vi "Device to String.vi"(11 "Devices":T1[](array[typedef])) -> (3 "delimited string":string)   [LabVIEW 2019, in "DAQmx.lvclass"]
uses:
  DAQmx.lvclass
  typedefs/DeviceInfo--Cluster.ctl
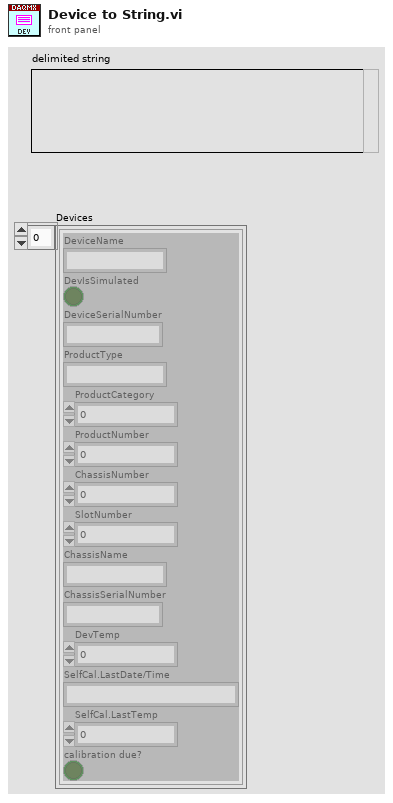
[diagram p1: front panel]
types:
  T1 = typedef "DAQmx.lvclass/DeviceInfo--Cluster.ctl" = cluster{"DeviceName":string, "DevIsSimulated":bool, "DeviceSerialNumber":string, "ProductType":string, "ProductCategory":i32, "ProductNumber":u32, "ChassisNumber":u32, "SlotNumber":u32, "ChassisName":string, "ChassisSerialNumber":string, "DevTemp":dbl, "SelfCal.LastDate/Time":string, "SelfCal.LastTemp":dbl, "calibration due?":bool}
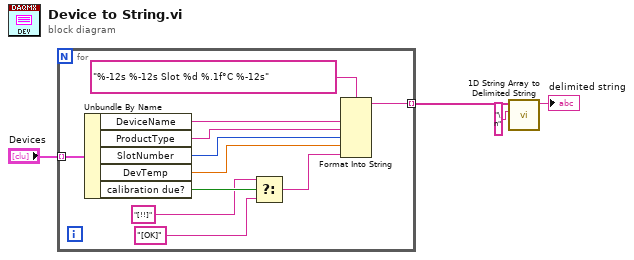
[diagram p0: block diagram]
diagram:
  n1 = for {
    tunnel: "Devices" -> [w15] mode=indexing
    tunnel: [w9] -> w1 mode=indexing
    n2 = Unbundle By Name(w15) -> ("DeviceName"=w10:string, "ProductType"=w13:string, "SlotNumber"=w12:u32, "DevTemp"=w11:dbl, "calibration due?"=w8:bool)
    n3 = Select(t="[!!]", s=w8, f="[OK]") -> (s? t:f=w7:string)
    n4 = Format Into String(format string="%-12s %-12s Slot %d %.1f°C %-12s", w10, w13, w12, w11, w7) -> (resulting string=w9:string)  [unwired: 2 in, 1 out]
  }
  n5 = call <vilib>:"1D String Array to Delimited String.vi"("delimiter"="\n", "string array"=w1) -> ("delimited string"=→"delimited string":string)  [unwired: 9 in]
